vi "FTW-ProjectItemManager-BroadcastMessage.vi"(0 "Project Item Manager":refnum<class "FTW-ProjectItemManager.lvclass">, 5 "Action Performed":string, 7 "Payload":variant, 11 "error in":errorcluster) -> (4 "Project Item Manager out":refnum<class "FTW-ProjectItemManager.lvclass">, 15 "error out":errorcluster)   [LabVIEW 2012, in "FTW-ProjectItemManager.lvclass"]
uses:
  FTW-ProjectItemManager.lvclass
  FTW-ProjectItemManager.lvclass/FTW-ProjectItemManager.ctl
  Core/Messaging/Messenger.Actor/FTW-Messenger-Actor.lvclass
panel:
  # "Inputs"
  # "Outputs"
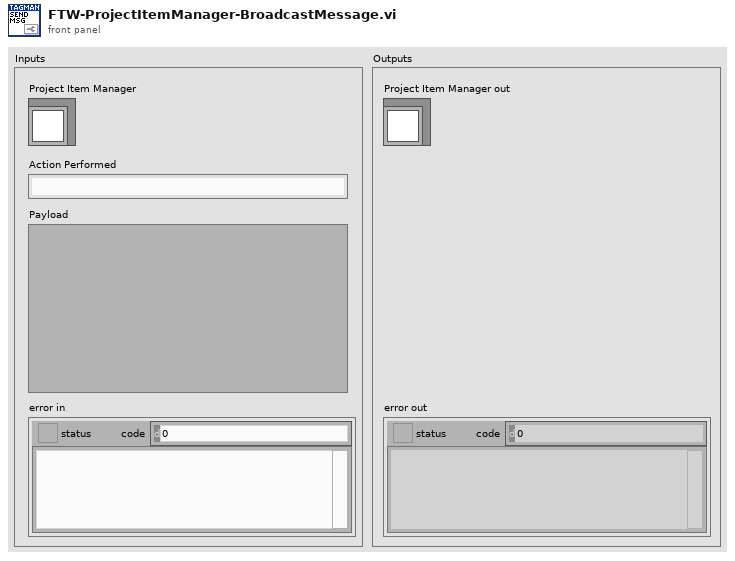
[diagram p1: front panel]
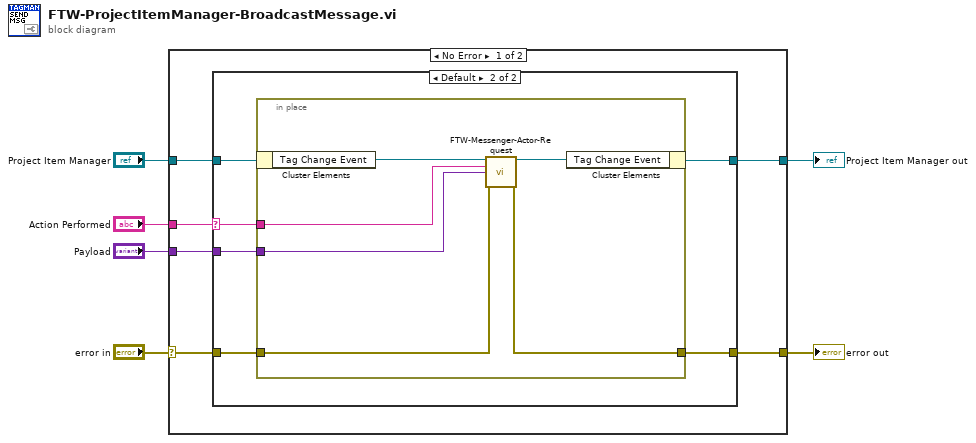
[diagram p0: block diagram]
diagram:
  n1 = case shown="No Error" "error in" {
    selector: "error in" -> [w10 w28]
    tunnel: [w9 w28] -> w6
    tunnel: [w12 w27] -> w4
    tunnel: "Project Item Manager" -> [w11 w27]
    tunnel: "Action Performed" -> [w7 _]
    tunnel: "Payload" -> [w8 _]
    frame No Error {
      n2 = case shown="Default" w7 {
        selector: w7 -> [_ w15]
        tunnel: [w14 w20] -> w12
        tunnel: w11 -> [w14 w19]
        tunnel: w10 -> [w13 w18]
        tunnel: [w13 w17] -> w9
        tunnel: w8 -> [_ w16]
        frame "" {
        }
        frame Default {
          n3 = in-place {
            in-place-border: [w24] -> w17
            in-place-border: w18 -> [w23]
            in-place-border: w15 -> [w22]
            in-place-border: w16 -> [w21]
            n4 = in-place-cluster #1(w19) -> ("Tag Change Event"=w26:refnum<class "FTW-Messenger-Actor.lvclass">)
            n5 = call-dynamic "FTW-Messenger-Actor-Request.vi"("Messenger"=w26, "Parameter"=w22, "Payload"=w21, "error in"=w23) -> ("Messenger out"=w25:refnum<class "FTW-Messenger-Actor.lvclass">, "error out"=w24:errorcluster)  [unwired: 10 in]
            n6 = in-place-cluster #1("Tag Change Event"=w25) -> (w20:refnum<class "FTW-ProjectItemManager.lvclass">)
          }
        }
      }
    }
    frame Error {
    }
  }
  "error out" <- w6
  "Project Item Manager out" <- w4
